vi "Validate Trigger Config.vi"(8 "error in (no error)":errorcluster, 11 "TriggerDelayControl in":refnum<class "TriggerDelayControl.lvclass">) -> (0 "error out":errorcluster, 3 "TriggerDelayControl out":refnum<class "TriggerDelayControl.lvclass">)   [LabVIEW 2020, in "VolatusControl.lvlib" / "TriggerDelayControl.lvclass"]
uses:
  TriggerDelayControl.lvclass
  TriggerDelayControl.lvclass/TriggerDelayControl.ctl
  Channel Type.ctl
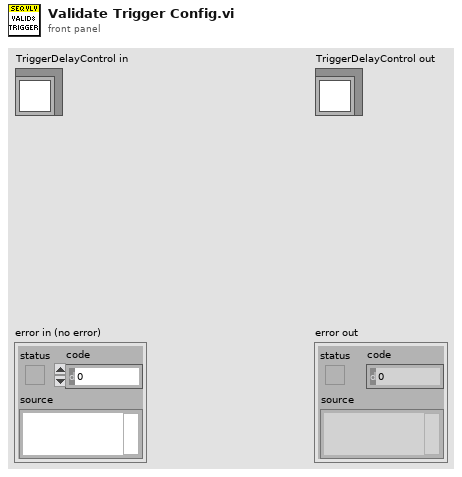
[diagram p1: front panel]
types:
  T1 = typedef "VolatusControl.lvlib/TriggerDelayControl.lvclass/Channel Type.ctl" = enum16{"Double", "String"}
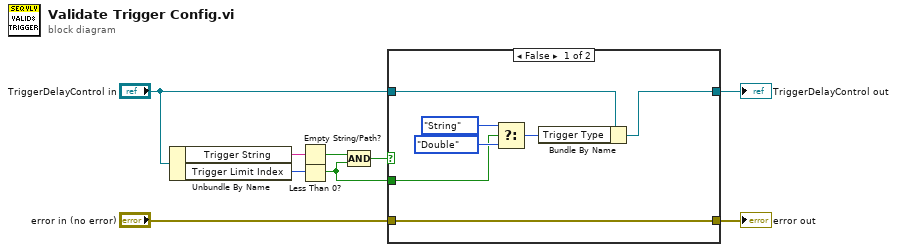
[diagram p0: block diagram]
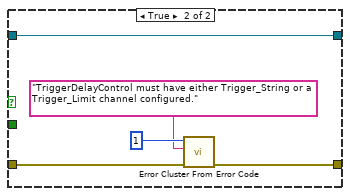
[diagram p2: hidden frame]
diagram:
  n1 = Unbundle By Name("TriggerDelayControl in") -> ("Trigger String"=w8:string, "Trigger Limit Index"=w9:i32)
  n2 = Empty String/Path?(string/path=w8) -> (empty?=w7:bool)
  n3 = Less Than 0?(x=w9) -> (x < 0?=w1:bool)
  n4 = Compound Arithmetic op=AND(w7, w1) -> (w6:bool)
  n5 = case shown="False" w6 {
    tunnel: "error in (no error)" -> [w16 w21]
    tunnel: [w16 w20] -> w4
    tunnel: "TriggerDelayControl in" -> [w15 w17]
    tunnel: [w14 w17] -> w2
    tunnel: w1 -> [w10 _]
    frame False {
      n6 = Select(t=Channel_Type."String" ("Trigger Type"), s=w10, f=Channel_Type."Double" ("Trigger Type")) -> (s? t:f=w11:T1)
      n7 = Bundle By Name(cluster=w15, "Trigger Type"=w11) -> (w14:refnum<class "TriggerDelayControl.lvclass">)
    }
    frame True {
      n8 = call <vilib>:"Error Cluster From Error Code.vi"("error in (no error)"=w21, "error message (\"\")"="TriggerDelayControl must have either Trigger_String or a Trigger_Limit channel configured.", "error code (0)"=1) -> ("error out"=w20:errorcluster)  [unwired: 6 in]
    }
  }
  "error out" <- w4
  "TriggerDelayControl out" <- w2
